vi "g-sugar-demo.vi"() -> ()   [LabVIEW 2020]
uses:
  94281f2b-890a-4e6d-a4f6-f467c7cae9bd.vi
  22db832c-b649-4559-a7c5-047596d71a6d.vi
  3d6616d8-2409-4fc6-9acc-faa54112bb19.vi
  eb25052e-2497-4765-bd5c-0c4d8bb99cef.vi
  ec6209c7-b53a-483d-9164-8fe77fea1447.vi
  715cf14a-5436-4b88-8b1e-78c662d2b827.vi
  3b77a937-6a2f-4878-9bc4-7f4bddd8323b.vi
  g-sugar.lvlib
  <vilib>/Analysis/NI_AALPro.lvlib
  33f22c91-7eff-4e5d-a32d-81f63ad906ef.vi
  519a8e68-bc07-43a2-981e-45f3fe44903d.vi
  4a577009-85e7-408d-aa54-6588ca8c41f8.vi
  30d617d3-d0e7-4e30-ab6e-2d342fca4c74.vi
  aa25d6cc-2931-477c-b6b3-9691ee10c1e4.vi
  e9cdb48e-78c8-4262-9879-220555bf7773.vi
  51ce616f-4567-4dbe-b0d1-12801dd102df.vi
  99fb4af5-680f-4626-9c76-18eb3f553bf0.vi
  85cc2e0d-3d79-4498-99a3-2fbd9174a0e7.vi
  <vilib>/ErrorRing/Error Ring.xnode
  68248d10-a314-448d-9c6a-9a330b4740aa.vi
  1d5c51dc-61f8-4fd2-bd84-5a3960a11abb.vi
  4b71f9a0-260f-46ca-bd72-54907fb75199.vi
  423ef1d7-39c7-482c-988b-842c3af334f1.vi
  d0fd2a03-687f-4279-b06c-406d47a19201.vi
  5947840f-00c0-44d2-8acd-1744f0fa6371.vi
  ee6e2a49-9c6d-4a08-84a9-3bd5615dd956.vi
  b232403f-50e3-4e97-8855-432ee40cb43d.vi
  d5dc5bf1-0620-422e-a9de-d0aecb74e2c8.vi
  792c066e-54cb-48e5-ae26-35e9aa0052d2.vi
  2cff2831-ec82-4b67-b912-af5035cf2bfa.vi
  e99b7bfd-0cfa-4cc0-8dd1-e3f468239a35.vi
  64a0e5fd-e8b8-4e95-948d-783c73bba6db.vi
  65d1c7ec-8a2d-480b-9861-fcfb9798beb0.vi
  83079c20-3910-436d-8488-6ed400462aac.vi
  45bf196d-d7b9-4f31-8bb8-42e6f8cb90b3.vi
  82b46934-9082-4ea7-b098-1d13be7c6a95.vi
  d85b58e6-5a10-4eed-a5dc-063cb5e64c46.vi
  b37acbe2-3c7a-42fe-b3c1-7b20d18f4c81.vi
  a485507d-2d7f-441e-aca8-16e1552411c8.vi
  bf0556a1-b16c-40cf-ae48-c400b6a0c3f9.vi
  4252a19e-cb24-4df5-b3ad-1eaafdbb9b5d.vi
  1b34461e-3e93-4e65-9fa3-404b33ffa90a.vi
  d828c4ad-8b35-4c2f-a3db-6a2b606c1c28.vi
  e48b0d5a-9f4f-4425-97f3-c9b64dce03a6.vi
  f9c1b5f8-e247-4c56-b062-eda7e1931e07.vi
  4811df1d-c4ac-45a0-8b7a-723235645d22.vi
  a602817d-79a6-4b8c-849a-5f13c7382d47.vi
  adbfa3d3-e960-405f-8091-50d5b080d598.vi
  4afd3748-bdc5-49c8-8b8d-0f13ded91422.vi
  d02df930-558f-41a8-bd33-d6e2823eb075.vi
  9e6ef8fc-4692-4657-bee1-be067bab3a07.vi
  fd33748e-e334-4565-8caf-3866f495208c.vi
  f4f2b763-330e-45c9-8ba8-adba11cec235.vi
  44106e74-6d40-4b07-a7fb-d67bb38b436d.vi
  8ba80f89-70fb-4c35-8445-d8927b049e74.vi
  a0894bde-2cb1-4ca8-830c-4f72b4038883.vi
panel:
  out "output 2":dbl[](array[numeric])
  out "duration s 2":dbl
  out "duration s":dbl
  out "timestamp out 3":timestamp format="%<%x %.3X>T"
  out "s? t:f":string
  out "value out 3":string
  out "set":set{i32[]}(c389)
  out "union 2":set{i32}(c389)
  out "union":set{i32}(c389)
  in  "chan list":string[](array[string])
  in  "input 1":string
  out "keys":i32[](array[numeric])
  in  "Array A":string[](array[string])=["0", "1", "2"]
  in  "Array B":i32[](array[numeric])=[0, 1, 2]
  in  "Array A":string[](array[string])=["0", "1", "2"]
  in  "Array B":i32[](array[numeric])=[0, 1, 2]
  in  "Array B":i32[](array[numeric])=[0, 1, 2]
  in  "Array A":string[](array[string])=["0", "1", "2"]
  out "map 2":map{string, dbl}(c390)
  out "map":map{string, dbl}(c390)
  out "output 5":errorcluster
  out "output 4":errorcluster
  out "value out 2":string[](array[string])
  out "value out":i32
  out "set 3":set{string}(c389)
  out "set 2":set{string}(c389)
  out "same size 3":bool
  out "same size 2":bool
  out "same size":bool
  out "output":dbl[](array[numeric])
  out "timestamp out 2":timestamp format="%<%x %.3X>T"
  out "timestamp out":timestamp format="%<%x %.3X>T"
  out "items":dbl[](array[numeric])
  out "keys":i32[](array[numeric])
  out "items":i32[](array[numeric])
  out "keys":string[](array[string])
  out "delimited string 3":string
  out "delimited string":string
  out "delimited string 2":string
  in  "array":string[](array[string])
  in  "delimiter":string="\t"
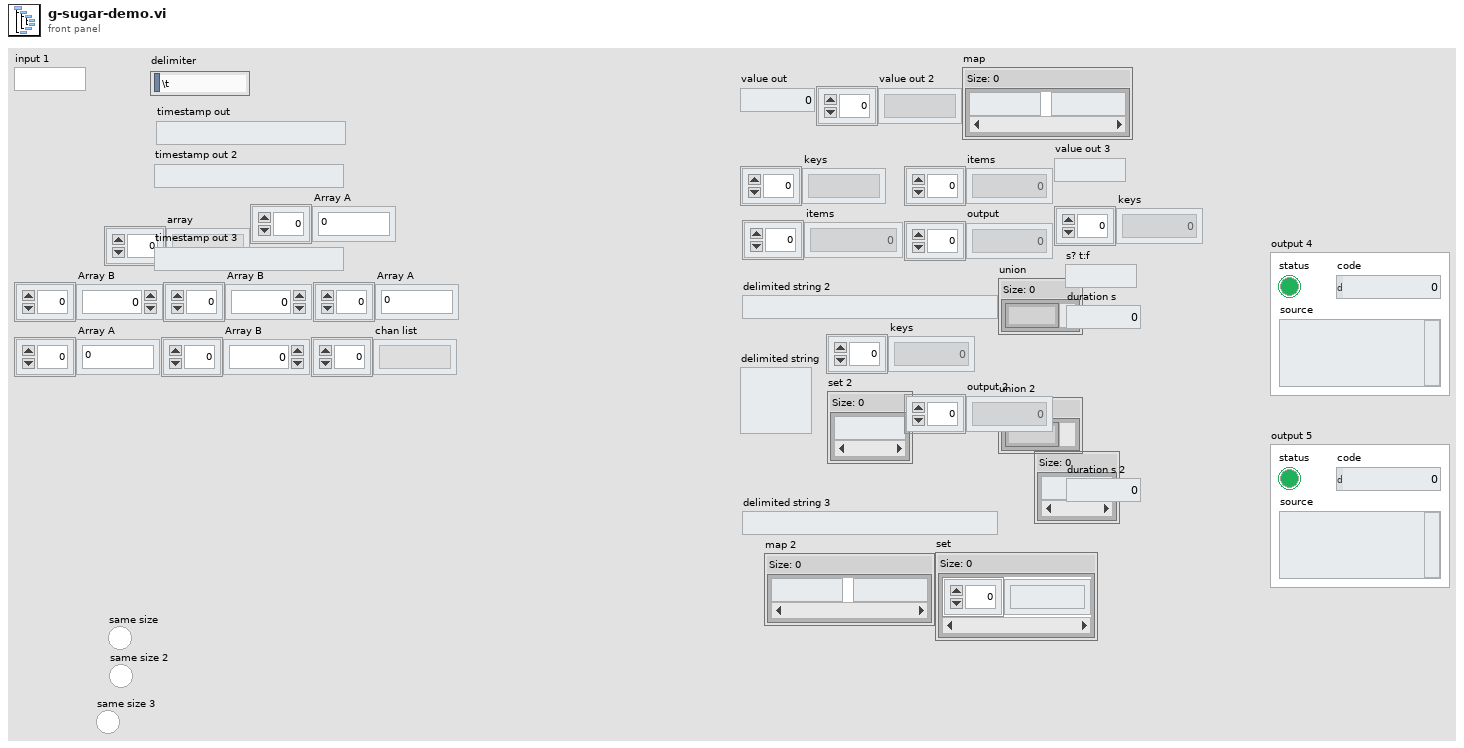
[diagram p1: front panel]
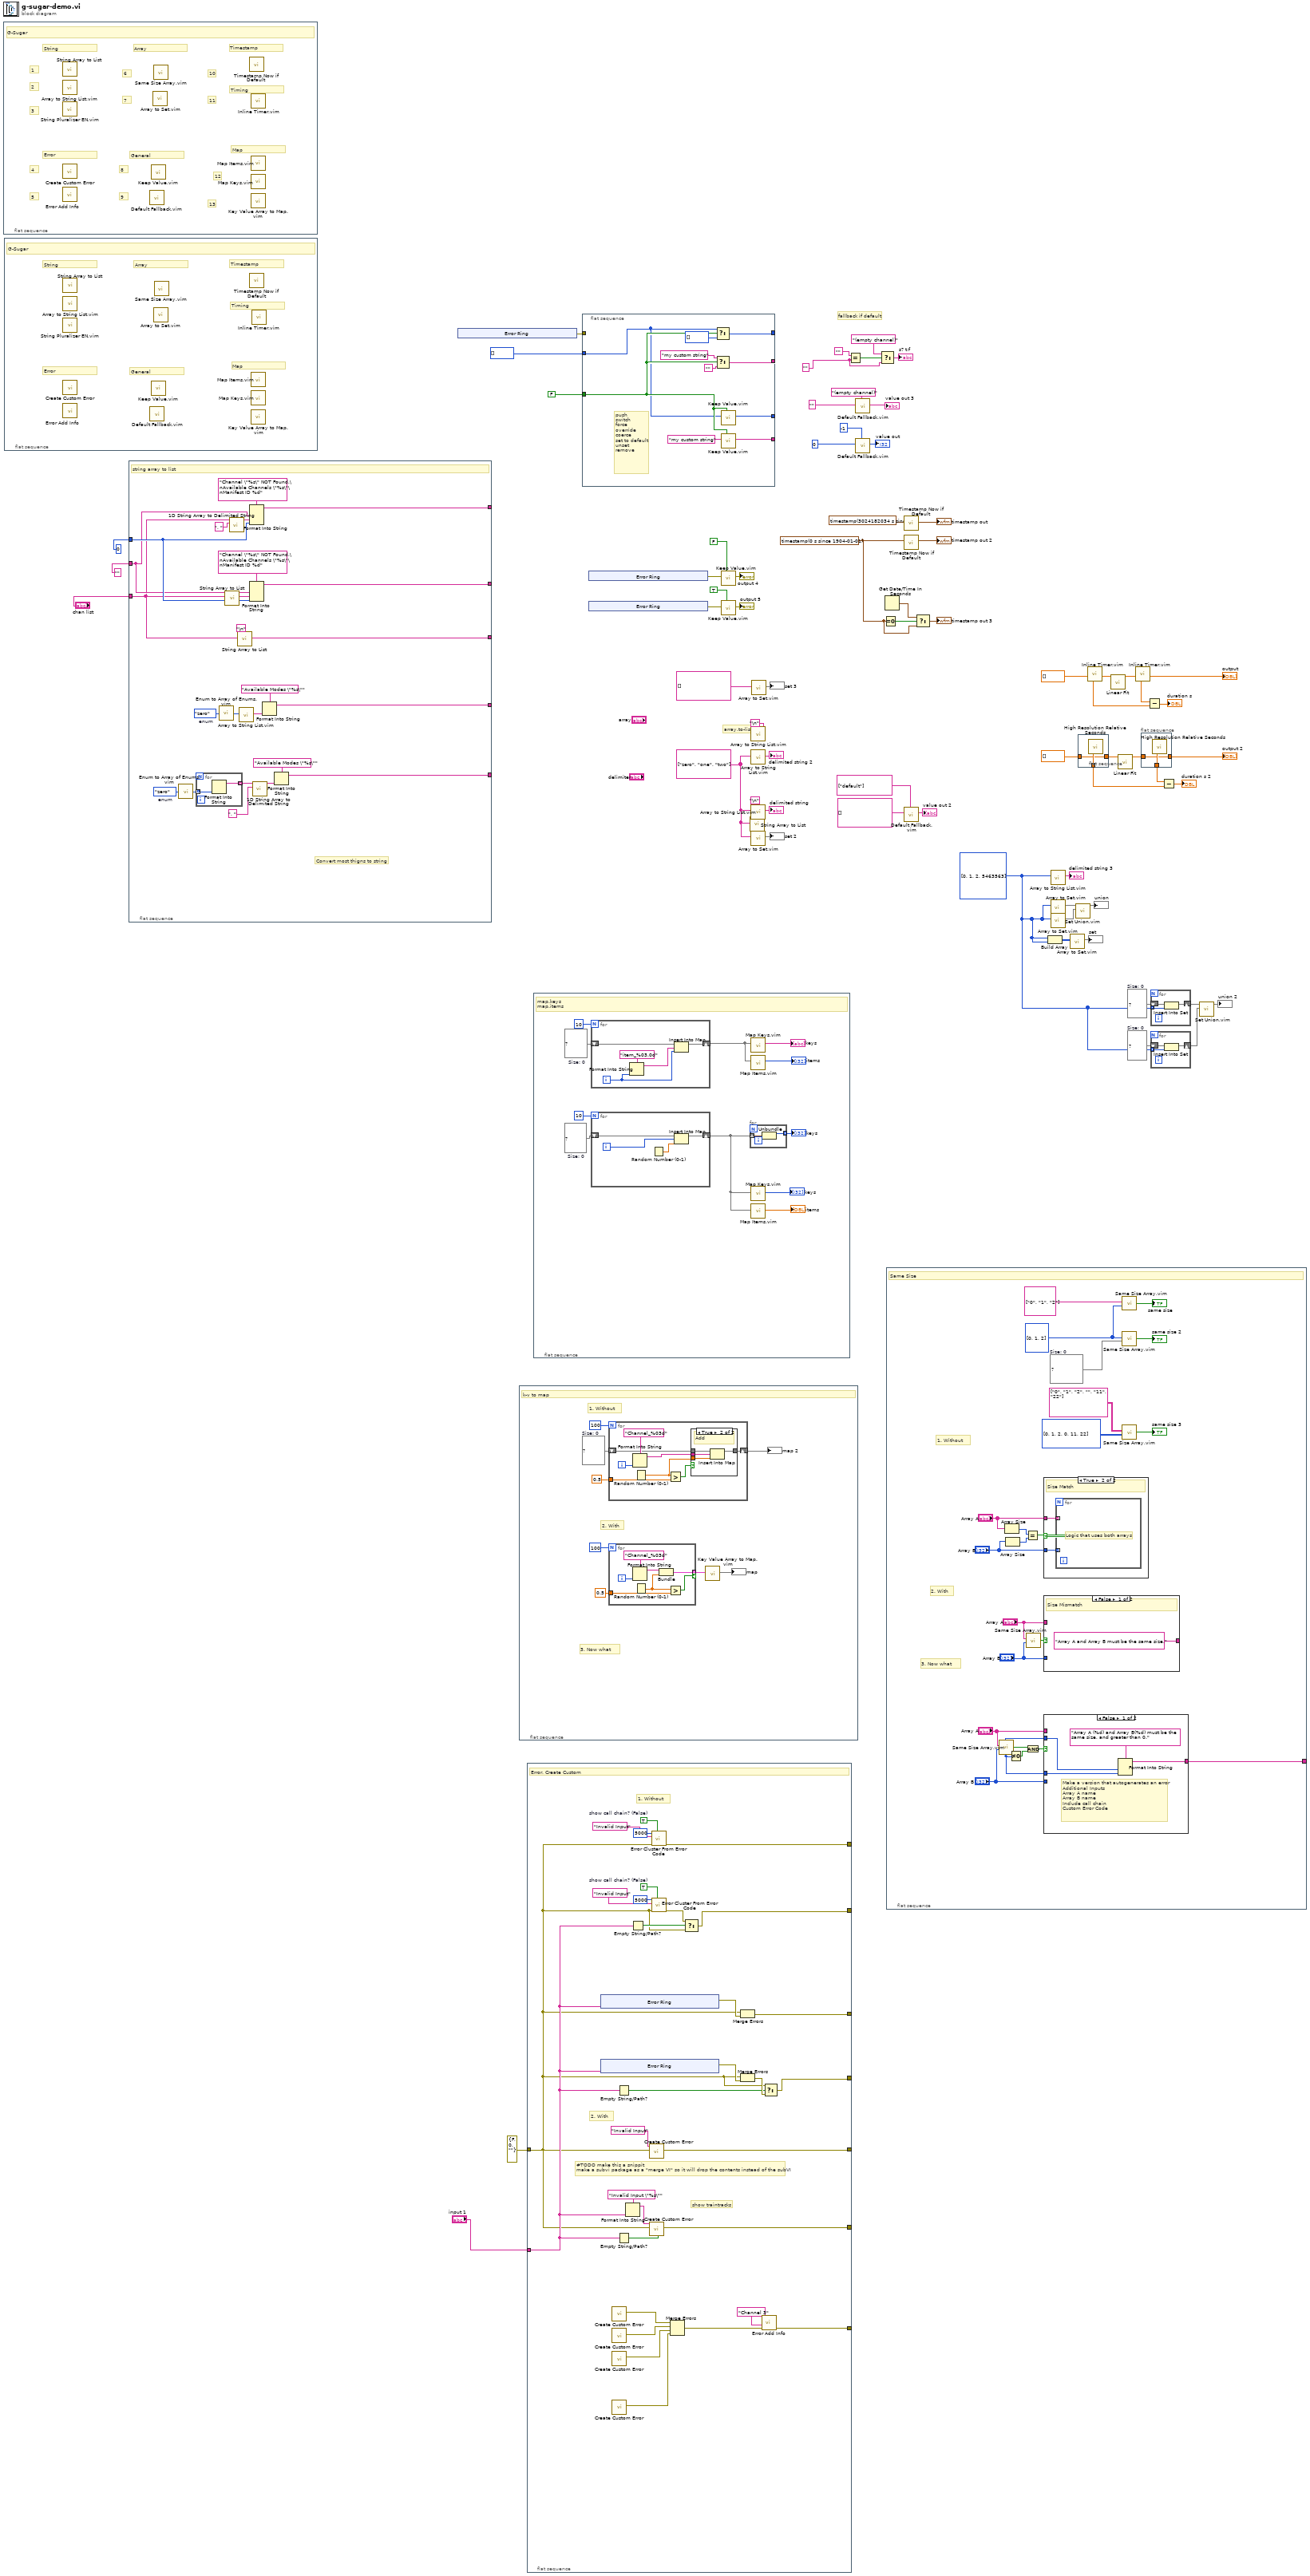
[diagram p0: block diagram]
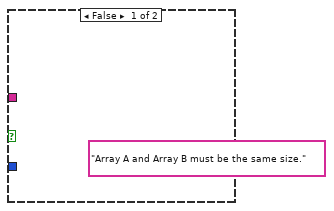
[diagram p3: hidden frame]
diagram:
  w14 = "" ("input 1")
  w27 = set{i32} {}  # Size: 0
  w30 = set{i32} {}  # Size: 0
  w10 = timestamp(0 s since 1904-01-01) ("Time Stamp")
  w25 = i32[] [0, 1, 2, 5463563]
  w41 = string[] ["zero", "one", "two"] ("array")
  # "fallback if default"
  # "array.to-list"
  n1 = flat-sequence {
    frame #0 {
      # "13"
      # "12"
      # "Map"
      # "11"
      # "10"
      # "Timing"
      # "Timestamp"
      # "9"
      # "8"
      # "General"
      # "7"
      # "6"
      # "Array"
      # "5"
      # "4"
      # "Error"
      # "3"
      # "2"
      # "1"
      # "String"
      # "G-Sugar"
      n2 = call "String Array to List.vi"() -> ()  [unwired: 11 in, 1 out]
      n3 = call "Array to String List.vim"() -> ()  [unwired: 11 in, 1 out]
      n4 = call "String Pluralizer EN.vim"() -> ()  [unwired: 11 in, 1 out]
      n5 = call "Create Custom Error.vi"() -> ()  [unwired: 11 in, 1 out]
      n6 = call "Error Add Info.vi"() -> ()  [unwired: 11 in, 1 out]
      n7 = call "Default Fallback.vim"() -> ()  [unwired: 10 in, 2 out]
      n8 = call "Keep Value.vim"() -> ()  [unwired: 9 in, 1 out]
      n9 = call "Array to Set.vim"() -> ()  [unwired: 11 in, 1 out]
      n10 = call "Same Size Array.vim"() -> ()  [unwired: 4 in, 3 out]
      n11 = call "Timestamp Now if Default.vi"() -> ()  [unwired: 11 in, 1 out]
      n12 = call "Map Items.vim"() -> ()  [unwired: 11 in, 1 out]
      n13 = call "Map Keys.vim"() -> ()  [unwired: 11 in, 1 out]
      n14 = call "Key Value Array to Map.vim"() -> ()  [unwired: 11 in, 1 out]
      n15 = call "Inline Timer.vim"() -> ()  [unwired: 8 in, 2 out]
    }
  }
  n16 = flat-sequence {
    frame #0 {
      # "Map"
      # "Timing"
      # "Timestamp"
      # "General"
      # "Array"
      # "Error"
      # "String"
      # "G-Sugar"
      n17 = call "String Array to List.vi"() -> ()  [unwired: 11 in, 1 out]
      n18 = call "Array to String List.vim"() -> ()  [unwired: 11 in, 1 out]
      n19 = call "String Pluralizer EN.vim"() -> ()  [unwired: 11 in, 1 out]
      n20 = call "Create Custom Error.vi"() -> ()  [unwired: 11 in, 1 out]
      n21 = call "Error Add Info.vi"() -> ()  [unwired: 11 in, 1 out]
      n22 = call "Default Fallback.vim"() -> ()  [unwired: 10 in, 2 out]
      n23 = call "Keep Value.vim"() -> ()  [unwired: 9 in, 1 out]
      n24 = call "Array to Set.vim"() -> ()  [unwired: 11 in, 1 out]
      n25 = call "Same Size Array.vim"() -> ()  [unwired: 4 in, 3 out]
      n26 = call "Timestamp Now if Default.vi"() -> ()  [unwired: 11 in, 1 out]
      n27 = call "Map Items.vim"() -> ()  [unwired: 11 in, 1 out]
      n28 = call "Map Keys.vim"() -> ()  [unwired: 11 in, 1 out]
      n29 = call "Key Value Array to Map.vim"() -> ()  [unwired: 11 in, 1 out]
      n30 = call "Inline Timer.vim"() -> ()  [unwired: 8 in, 2 out]
    }
  }
  n31 = flat-sequence {
    tunnel: [w91] -> _
    tunnel: "chan list" -> [w83]
    tunnel: [w87] -> _
    tunnel: 0 -> [w86]
    tunnel: "" ("input 1") -> [w85]
    tunnel: [w82] -> _
    tunnel: [w77] -> _
    tunnel: [w70] -> _
    frame #0 {
      w74 = enum16{"zero", "one", "two", "three"}."zero"  # enum
      w80 = enum16{"zero", "one", "two", "three"}."zero"  # enum
      # "Convert most thigns to string"
      # "string array to list"
      n32 = call "Enum to Array of Enums.vim"("enum"=w74) -> ("array of enums"=w73:enum16{"zero", "one", "two", "three"}[])
      n33 = for {
        tunnel: w73 -> [w95] mode=indexing
        tunnel: [w94] -> w71 mode=indexing
        n34 = Format Into String(w95) -> (resulting string=w94:string)  [unwired: 3 in, 1 out]
      }
      n35 = call "Enum to Array of Enums.vim"("enum"=w80) -> ("array of enums"=w81:enum16{"zero", "one", "two", "three"}[])
      n36 = call "String Array to List.vi"("string array"=w83) -> ("delimited string"=w92:string)  [unwired: 10 in]
      n37 = call <vilib>:"1D String Array to Delimited String.vi"("delimiter"=", " ("delimiter (, )"), "string array"=w83) -> ("delimited string"=w90:string)  [unwired: 9 in]
      n38 = call "String Array to List.vi"("delimiter (, )"="\n", "string array"=w83) -> ("delimited string"=w82:string)  [unwired: 9 in]
      n39 = call "Array to String List.vim"("array"=w81) -> ("delimited string"=w78:string)  [unwired: 10 in]
      n40 = Format Into String(format string="Channel \"%s\" NOT Found.\nAvailable Channels \"%s\"\nManifest ID %d", w85, w90, w86) -> (resulting string=w87:string)  [unwired: 2 in, 1 out]
      n41 = Format Into String(format string="Channel \"%s\" NOT Found.\nAvailable Channels \"%s\"\nManifest ID %d", w85, w92, w86) -> (resulting string=w91:string)  [unwired: 2 in, 1 out]
      n42 = call <vilib>:"1D String Array to Delimited String.vi"("delimiter"=", " ("delimiter (, )"), "string array"=w71) -> ("delimited string"=w76:string)  [unwired: 9 in]
      n43 = Format Into String(format string="Available Modes \"%s\"", w78) -> (resulting string=w77:string)  [unwired: 2 in, 1 out]
      n44 = Format Into String(format string="Available Modes \"%s\"", w76) -> (resulting string=w70:string)  [unwired: 2 in, 1 out]
    }
  }
  n45 = xnode "Error Ring"() -> ("error out"=w22:errorcluster)
  n46 = flat-sequence {
    frame #0 {
      w97 = map{string, dbl} {}  # Size: 0
      # "3. Now what"
      # "2. With"
      # "1. Without"
      # "k-v to map"
      n47 = for {
        N: 100 -> [_]
        tunnel: 0.5 ("y") -> [w109]
        shift-right: [w105] -> w96
        shift-left: w97 -> [w107]
        i -> [w110]
        n48 = Format Into String(format string="Channel_%03d", w110) -> (resulting string=w108:string)  [unwired: 2 in, 1 out]
        n49 = Random Number (0-1)() -> (number: 0 to 1=w106:dbl)
        n50 = Greater?(x=w106, y=w109) -> (0:w104:bool)
        n51 = case shown="True" w104 {
          tunnel: w108 -> [_ w116]
          tunnel: w107 -> [w112 w115]
          tunnel: w106 -> [_ w114]
          tunnel: [w112 w113] -> w105
          frame False {
            # "Don't Add"
          }
          frame True {
            # "Add"
            n52 = Insert Into Map(map in=w115, key=w116, value=w114) -> (map out=w113:map{string, dbl})  [unwired: 2 out]
          }
        }
      }
      "map 2" <- w96
      n53 = for {
        N: 100 -> [_]
        tunnel: 0.5 ("y") -> [w119]
        tunnel: [w118] -> w101 mode=indexing if=w117
        i -> [w122]
        n54 = Format Into String(format string="Channel_%03d", w122) -> (resulting string=w121:string)  [unwired: 2 in, 1 out]
        n55 = Random Number (0-1)() -> (number: 0 to 1=w120:dbl)
        n56 = Bundle(w121, "number: 0 to 1"=w120) -> (w118:cluster{string, "number: 0 to 1":dbl})  [unwired: 1 in]
        n57 = Greater?(x=w120, y=w119) -> (0:w117:bool)
      }
      n58 = call "Key Value Array to Map.vim"("key value array"=w101) -> ("map"=→"map":map{string, dbl})  [unwired: 10 in]
    }
  }
  n59 = flat-sequence {
    tunnel: errorcluster {"status"=FALSE, "code"=0, "source"=""} ("upstream error") -> [w135]
    tunnel: [w148] -> _
    tunnel: "input 1" -> [w138]
    tunnel: [w144] -> _
    tunnel: [w142] -> _
    tunnel: [w139] -> _
    tunnel: [w134] -> _
    tunnel: [w131] -> _
    tunnel: [w124] -> _
    frame #0 {
      w147 = TRUE  # show call chain? (False)
      w151 = TRUE  # show call chain? (False)
      # "#TODO make this a snippit\nmake a subvi package as a \"merge VI\" so it will drop the contents instead of the subVI"
      # "show traintracks"
      # "2. With"
      # "1. Without"
      # "Error. Create Custom"
      n60 = xnode "Error Ring"("parameter 0"=w138) -> ("error out"=w143:errorcluster)
      n61 = xnode "Error Ring"("parameter 0"=w138) -> ("error out"=w141:errorcluster)
      n62 = call "Create Custom Error.vi"() -> ("error out"=w130:errorcluster)  [unwired: 11 in]
      n63 = call "Create Custom Error.vi"() -> ("error out"=w129:errorcluster)  [unwired: 11 in]
      n64 = call "Create Custom Error.vi"() -> ("error out"=w128:errorcluster)  [unwired: 11 in]
      n65 = call "Create Custom Error.vi"() -> ("error out"=w127:errorcluster)  [unwired: 11 in]
      n66 = Empty String/Path?(string/path=w138) -> (empty?=w137:bool)
      n67 = Empty String/Path?(string/path=w138) -> (empty?=w132:bool)
      n68 = Format Into String(format string="Invalid Input \"%s\"" ("error message"), w138) -> (resulting string=w133:string)  [unwired: 2 in, 1 out]
      n69 = Empty String/Path?(string/path=w138) -> (empty?=w150:bool)
      n70 = call "Create Custom Error.vi"("error in"=w135, "error message"="Invalid Input") -> ("error out"=w134:errorcluster)  [unwired: 9 in]
      n71 = call "Create Custom Error.vi"("enable (T)"=w132, "error in"=w135, "error message"=w133) -> ("error out"=w131:errorcluster)  [unwired: 8 in]
      n72 = call <vilib>:"Error Cluster From Error Code.vi"("show call chain? (False)"=w147, "error in (no error)"=w135, "error message (\"\")"="Invalid Input" ("error message"), "error code (0)"=5000) -> ("error out"=w144:errorcluster)  [unwired: 5 in]
      n73 = call <vilib>:"Error Cluster From Error Code.vi"("show call chain? (False)"=w151, "error in (no error)"=w135, "error message (\"\")"="Invalid Input" ("error message"), "error code (0)"=5000) -> ("error out"=w149:errorcluster)  [unwired: 5 in]
      n74 = Merge Errors(w130, w129, w128, w127) -> (w126:errorcluster)
      n75 = Select(t=w149, s=w150, f=w135) -> (s? t:f=w148:errorcluster)
      n76 = Merge Errors(w135, w143) -> (w142:errorcluster)
      n77 = Merge Errors(w135, w141) -> (w140:errorcluster)
      n78 = call "Error Add Info.vi"("error in"=w126, "Info"="Channel 3") -> ("error out"=w124:errorcluster)  [unwired: 9 in]
      n79 = Select(t=w135, s=w137, f=w140) -> (s? t:f=w139:errorcluster)
    }
  }
  n80 = flat-sequence {
    frame #0 {
      w174 = map{i32, dbl} {}  # Size: 0
      w178 = map{string, i32} {}  # Size: 0
      # "map.keys\nmap.items"
      n81 = for {
        N: 10 -> [_]
        shift-right: [w183] -> w176
        shift-left: w178 -> [w182]
        i -> [w184]
        n82 = Format Into String(format string="item_%03.0d", w184) -> (resulting string=w185:string)  [unwired: 2 in, 1 out]
        n83 = Insert Into Map(map in=w182, key=w185, value=w184) -> (map out=w183:map{string, i32})  [unwired: 2 out]
      }
      n84 = for {
        N: 10 -> [_]
        shift-right: [w190] -> w170
        shift-left: w174 -> [w189]
        i -> [w188]
        n85 = Random Number (0-1)() -> (number: 0 to 1=w187:dbl)
        n86 = Insert Into Map(map in=w189, key=w188, value=w187) -> (map out=w190:map{i32, dbl})  [unwired: 2 out]
      }
      n87 = for {
        tunnel: w170 -> [w181] mode=indexing
        tunnel: [w180] -> w169 mode=indexing
        n88 = Unbundle(w181) -> (w180:i32)  [unwired: 1 out]
      }
      "keys" <- w169
      n89 = call "Map Keys.vim"("map"=w176) -> ("keys"=→"keys":string[])  [unwired: 10 in]
      n90 = call "Map Items.vim"("map"=w176) -> ("items"=→"items":i32[])  [unwired: 10 in]
      n91 = call "Map Keys.vim"("map"=w170) -> ("keys"=→"keys":i32[])  [unwired: 10 in]
      n92 = call "Map Items.vim"("map"=w170) -> ("items"=→"items":dbl[])  [unwired: 10 in]
    }
  }
  n93 = flat-sequence {
    tunnel: FALSE ("keep input?") -> [w192]
    tunnel: [w197] -> _
    tunnel: [w196] -> _
    tunnel: [w195] -> _
    tunnel: w22 -> [_]
    tunnel: i32[] [] -> [w191]
    tunnel: [w193] -> _
    frame #0 {
      # "push\nswitch\nforce\noverride\ncoerce\nset to default\nunset\nremove"
      n94 = Select(t=w191, s=w192, f=i32[] []) -> (s? t:f=w193:i32[])
      n95 = Select(t="my custom string" ("input 1"), s=w192, f="") -> (s? t:f=w195:string)
      n96 = call "Keep Value.vim"("keep input?"=w192, "input"=w191) -> ("output"=w197:i32[])  [unwired: 7 in]
      n97 = call "Keep Value.vim"("keep input?"=w192, "input"="my custom string" ("input 1")) -> ("output"=w196:string)  [unwired: 7 in]
    }
  }
  n98 = xnode "Error Ring"() -> ("error out"=w47:errorcluster)
  n99 = xnode "Error Ring"() -> ("error out"=w42:errorcluster)
  n100 = call "Keep Value.vim"("keep input?"=FALSE, "input"=w47) -> ("output"=→"output 4":errorcluster)  [unwired: 7 in]
  n101 = call "Keep Value.vim"("keep input?"=TRUE, "input"=w42) -> ("output"=→"output 5":errorcluster)  [unwired: 7 in]
  n102 = call "String Array to List.vi"("string array"=w41) -> ()  [unwired: 10 in, 1 out]
  n103 = call "Array to String List.vim"("delimiter (, )"="\n") -> ()  [unwired: 10 in, 1 out]
  n104 = call "Array to String List.vim"("array"=w41) -> ("delimited string"=→"delimited string 2":string)  [unwired: 10 in]
  n105 = call "Array to String List.vim"("delimiter (, )"="\n", "array"=w41) -> ("delimited string"=→"delimited string":string)  [unwired: 9 in]
  n106 = call "Array to Set.vim"("array"=w41) -> ("set"=→"set 2":set{string})  [unwired: 10 in]
  n107 = call "Array to Set.vim"("array"=string[] []) -> ("set"=→"set 3":set{string})  [unwired: 10 in]
  n108 = Equal?(x="", y=w14) -> (x = y?=w16:bool)
  n109 = call "Default Fallback.vim"("fallback value (if default)"="(empty channel)" ("input 1"), "value"="" ("input 1")) -> ("value out"=→"value out 3":string)  [unwired: 8 in, 1 out]
  n110 = call "Default Fallback.vim"("fallback value (if default)"=-1, "value"=0) -> ("value out"=→"value out":i32)  [unwired: 8 in, 1 out]
  n111 = Select(t="(empty channel)" ("input 1"), s=w16, f=w14) -> (s? t:f=→"s? t:f":string)
  n112 = Equal To 0?(x=w10) -> (x = 0?=w11:bool)
  n113 = Get Date/Time In Seconds() -> (seconds since 1Jan1904=w12:timestamp)
  n114 = flat-sequence {
    tunnel: [w201] -> _
    frame #0 {
      w223 = set{string} {}  # Size: 0
      w219 = i32[] [0, 1, 2]
      # "3. Now what"
      # "2. With"
      # "1. Without"
      # "Same Size"
      n115 = call "Same Size Array.vim"("input 2"="Array B", "input 1"="Array A") -> ("same size?"=w211:bool, "size 2"=w215:i32, "size 1"=w214:i32)  [unwired: 2 in]
      n116 = Array Size(array="Array A") -> (size(s)=w203:i32)
      n117 = Array Size(array="Array B") -> (size(s)=w204:i32)
      n118 = Not Equal To 0?(x=w215) -> (x != 0?=w212:bool)
      n119 = Equal?(x=w203, y=w204) -> (x = y?=w207:bool)
      n120 = call "Same Size Array.vim"("input 2"="Array B", "input 1"="Array A") -> ("same size?"=w208:bool)  [unwired: 2 in, 2 out]
      n121 = And(x=w211, y=w212) -> (x .and. y?=w213:bool)
      n122 = case shown="True" w207 {
        tunnel: "Array A" -> [_ w226]
        tunnel: "Array B" -> [_ w225]
        frame False {
          (unwired) "Array A and Array B must be the same size." ("format string")
        }
        frame True {
          # "Size Match"
          n123 = for {
            tunnel: w226 -> [_] mode=indexing
            tunnel: w225 -> [_] mode=indexing
            # "Logic that uses both arrays"
          }
        }
      }
      n124 = case shown="False" w208 {
        tunnel: "Array A" -> [_ w235]
        tunnel: "Array B" -> [_ w234]
        tunnel: ["Array A and Array B must be the same size." ("format string") _] -> _
        frame False {
          # "Size Mismatch"
        }
        frame True {
          n125 = for {
            tunnel: w235 -> [_] mode=indexing
            tunnel: w234 -> [_] mode=indexing
            # "Logic that uses both arrays"
          }
        }
      }
      n126 = case shown="False" w213 {
        tunnel: "Array A" -> [_ w232]
        tunnel: "Array B" -> [_ w231]
        tunnel: w214 -> [w229 _]
        tunnel: w215 -> [w228 _]
        tunnel: [w227 _] -> w201
        frame False {
          # "Make a version that autogenerates an error\nAdditional Inputs\nArray A name\nArray B name\nInclude call chain\nCustom Error Code"
          n127 = Format Into String(format string="Array A (%d) and Array B(%d) must be the same size, and greater than 0.", w229, w228) -> (resulting string=w227:string)  [unwired: 2 in, 1 out]
        }
        frame True {
          n128 = for {
            tunnel: w232 -> [_] mode=indexing
            tunnel: w231 -> [_] mode=indexing
            # "Logic that uses both arrays"
          }
        }
      }
      n129 = call "Same Size Array.vim"("input 2"=w219, "input 1"=string[] ["0", "1", "2"]) -> ("same size?"=→"same size":bool)  [unwired: 2 in, 2 out]
      n130 = call "Same Size Array.vim"("input 2"=w223, "input 1"=w219) -> ("same size?"=→"same size 2":bool)  [unwired: 2 in, 2 out]
      n131 = call "Same Size Array.vim"("input 2"=i32[][] [[0, 1, 2], [0, 11, 22]], "input 1"=string[][] [["0", "1", "2"], ["", "11", "22"]]) -> ("same size?"=→"same size 3":bool)  [unwired: 2 in, 2 out]
    }
  }
  n132 = call "Timestamp Now if Default.vi"("timestamp in"=timestamp(3024182034.69 s since 1904-01-01) ("Time Stamp")) -> ("timestamp out"=→"timestamp out":timestamp)  [unwired: 10 in]
  n133 = call "Timestamp Now if Default.vi"("timestamp in"=w10) -> ("timestamp out"=→"timestamp out 2":timestamp)  [unwired: 10 in]
  n134 = call "Default Fallback.vim"("fallback value (if default)"=string[] ["default"] ("array"), "value"=string[] [] ("array")) -> ("value out"=→"value out 2":string[])  [unwired: 8 in, 1 out]
  n135 = Select(t=w12, s=w11, f=w10) -> (s? t:f=→"timestamp out 3":timestamp)
  n136 = Build Array(w25, w25) -> (w29:i32[][])
  n137 = call "Array to String List.vim"("array"=w25) -> ("delimited string"=→"delimited string 3":string)  [unwired: 10 in]
  n138 = call "Array to Set.vim"("array"=w25) -> ("set"=w34:set{i32})  [unwired: 10 in]
  n139 = call "Array to Set.vim"("array"=w25) -> ("set"=w33:set{i32})  [unwired: 10 in]
  n140 = call "Array to Set.vim"("array"=w29) -> ("set"=→"set":set{i32[]})  [unwired: 10 in]
  n141 = call "Set Union.vim"("set 2"=w33, "set 1"=w34) -> ("union"=→"union":set{i32})  [unwired: 9 in]
  n142 = flat-sequence {
    tunnel: [w237] -> w6
    tunnel: [w236] -> w5
    tunnel: dbl[] [] ("Y") -> [w236]
    frame #0 {
      n143 = call <vilib>:"High Resolution Relative Seconds.vi"() -> ("relative seconds"=w237:dbl)
    }
  }
  n144 = call "Inline Timer.vim"("input"=dbl[] [] ("Y")) -> ("output"=w59:dbl[], "relative seconds"=w62:dbl)  [unwired: 7 in]
  n145 = call <vilib>:"Linear Fit.vi"("Y"=w59) -> ("Best Linear Fit"=w58:dbl[])  [unwired: 10 in, 4 out]
  n146 = call <vilib>:"Linear Fit.vi"("Y"=w5) -> ("Best Linear Fit"=w3:dbl[])  [unwired: 10 in, 4 out]
  n147 = call "Inline Timer.vim"("input"=w58) -> ("output"=→"output":dbl[], "relative seconds"=w61:dbl)  [unwired: 7 in]
  n148 = flat-sequence {
    tunnel: [w239] -> w1
    tunnel: [w238] -> w2
    tunnel: w3 -> [w238]
    frame #0 {
      n149 = call <vilib>:"High Resolution Relative Seconds.vi"() -> ("relative seconds"=w239:dbl)
    }
  }
  n150 = Subtract(x=w61, y=w62) -> (x-y=→"duration s":dbl)
  n151 = for {
    shift-right: [w241] -> w26
    shift-left: w27 -> [w242]
    tunnel: w25 -> [w240] mode=indexing
    n152 = Insert Into Set(10:w240, 11:w242) -> (3:w241:set{i32})  [unwired: 1 out]
  }
  n153 = for {
    shift-right: [w244] -> w24
    shift-left: w30 -> [w245]
    tunnel: w25 -> [w243] mode=indexing
    n154 = Insert Into Set(10:w243, 11:w245) -> (3:w244:set{i32})  [unwired: 1 out]
  }
  n155 = Subtract(x=w1, y=w6) -> (x-y=→"duration s 2":dbl)
  n156 = call "Set Union.vim"("set 2"=w24, "set 1"=w26) -> ("union"=→"union 2":set{i32})  [unwired: 9 in]
  "output 2" <- w2
